vi "AIselector.vi"(8 "I/O element":T1(ring)) -> (3 "value":i16)   [LabVIEW 2014]
uses:
  <vilib>/rvi/eio/common/nirviEmuTemplateMethod_errors.vi
  <vilib>/eio/EIONode/EIONode.xnode
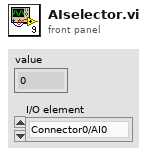
[diagram p1: front panel]
types:
  T1 = enum16{"Connector0/AI0", "Connector0/AI1", "Connector0/AI2", "Connector0/AI3", "Connector0/AI4", "Connector0/AI5", "Connector0/AI6", "Connector0/AI7"}
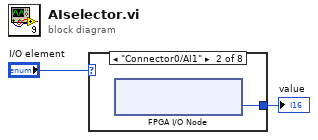
[diagram p0: block diagram]
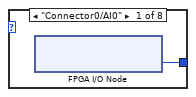
[diagram p2: hidden frame]
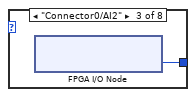
[diagram p3: hidden frame]
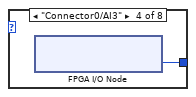
[diagram p4: hidden frame]
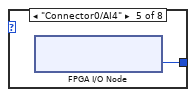
[diagram p5: hidden frame]
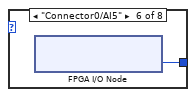
[diagram p6: hidden frame]
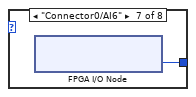
[diagram p7: hidden frame]
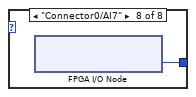
[diagram p8: hidden frame]
diagram:
  n1 = case shown="\"Connector0/AI1\"" "I/O element" {
    tunnel: [w3 w4 w5 w6 w7 w8 w9 w10] -> w1
    frame "Connector0/AI0" {
      n2 = xnode "FPGA I/O Node"() -> ("Connector0/AI0"=w3:i16)  [unwired: 1 in, 1 out]
    }
    frame "Connector0/AI1" {
      n3 = xnode "FPGA I/O Node"() -> ("Connector0/AI1"=w4:i16)  [unwired: 1 in, 1 out]
    }
    frame "Connector0/AI2" {
      n4 = xnode "FPGA I/O Node"() -> ("Connector0/AI2"=w5:i16)  [unwired: 1 in, 1 out]
    }
    frame "Connector0/AI3" {
      n5 = xnode "FPGA I/O Node"() -> ("Connector0/AI3"=w6:i16)  [unwired: 1 in, 1 out]
    }
    frame "Connector0/AI4" {
      n6 = xnode "FPGA I/O Node"() -> ("Connector0/AI4"=w7:i16)  [unwired: 1 in, 1 out]
    }
    frame "Connector0/AI5" {
      n7 = xnode "FPGA I/O Node"() -> ("Connector0/AI5"=w8:i16)  [unwired: 1 in, 1 out]
    }
    frame "Connector0/AI6" {
      n8 = xnode "FPGA I/O Node"() -> ("Connector0/AI6"=w9:i16)  [unwired: 1 in, 1 out]
    }
    frame "Connector0/AI7" {
      n9 = xnode "FPGA I/O Node"() -> ("Connector0/AI7"=w10:i16)  [unwired: 1 in, 1 out]
    }
  }
  "value" <- w1
